vi "PH_Beckhoff_StepMot.set modified data.vi"(0 "i ref in":refnum<vi>, 2 "i attribute":T1, 5 "error in (no error)":errorcluster) -> (14 "i ref out":refnum<vi>, 19 "error out":errorcluster)   [LabVIEW 2014, in "PH_Beckhoff_StepMot.lvlib"]
doc: "Writes the data into the attribute of an object. Then, the attribute dara are unlocked using the \"release\" method. Prior to calling THIS method, the attribute data must have been locked using the methods \"lock\" or \"get data to modify\".\n\n\nLicense Agreement for this software:\n\nCopyright (C)\nGesellschaft für Schwerionenforschung, GSI\nPlanckstr. 1\n64291 Darmstadt\nGermany\n\nContact: D.Beck@gsi.de \n\nThis program is free software; you can redistribute it and/or modify it under the terms of the GNU General Public License as published by the Free Software Foundation; either version 2 of the license, or (at your option) any later version.\n\nThis program is distributed in the hope that it will be useful, but WITHOUT ANY WARRANTY; without even the implied warranty of MERCHANTABILITY or FITNESS FOR A PARTICULAR PURPOSE. See the GNU General License for more details (http://www.gnu.org).\n\nGesellschaft für Schwerionenforschung, GSI\nPlanckstr. 1, 64291 Darmstadt, Germany\nFor all questions and ideas contact: M.Richter@gsi.de, H.Brand@gsi.de or D.Beck@gsi.de.\nLast update: 17-JUN-2004"
uses:
  PH_Beckhoff_StepMot.lvlib
  PH_Beckhoff_StepMot.i attribute.ctl
  PH_Beckhoff_StepMot.Axis Cluster.ctl
  instr.lib/Beckhoff/Specials/Step Motor Klemmen/Beckhoff.Step Motor - Motor Configuration.ctl
  instr.lib/Beckhoff/Read and Write Register/Step Motor Klemmen/Beckhoff.Step Motor - Feature Register 1.ctl
  instr.lib/Beckhoff/Read and Write Register/Step Motor Klemmen/Beckhoff.Step Motor - Feature Register 2.ctl
  CS_Core/CSObj/CSObj.lvlib
  instr.lib/Beckhoff/Beckhoff - Driver np.lvlib
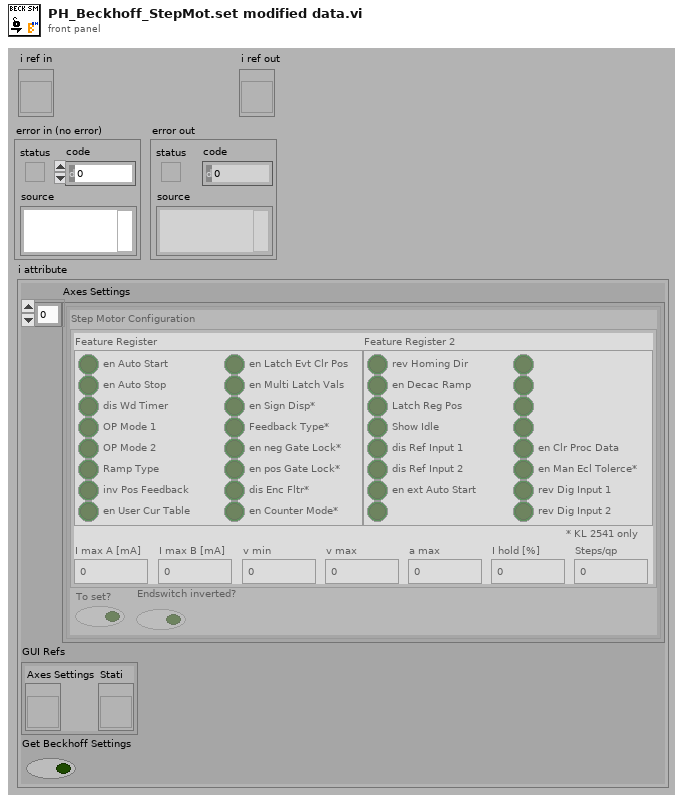
[diagram p1: front panel]
types:
  T1 = typedef "PH_Beckhoff_StepMot.lvlib/PH_Beckhoff_StepMot.i attribute.ctl" = cluster{"Axes Settings":T2[], "GUI Refs":cluster{"Axes Settings":refnum<vi>, "Stati":refnum<vi>}, "Get Beckhoff Settings":bool}
  T2 = typedef "PH_Beckhoff_StepMot.lvlib/PH_Beckhoff_StepMot.Axis Cluster.ctl" = cluster{"Step Motor Configuration":T3, "To set?":bool, "Endswitch inverted?":bool}
  T3 = typedef "Beckhoff - Driver np.lvlib/Beckhoff.Step Motor - Motor Configuration.ctl" = cluster{"Feature Register":T4, "I max A [mA]":dbl, "I max B [mA]":dbl, "v min":u32, "v max":u32, "a max":u32, "I hold [%]":u32, "Steps/qp":u32, "Feature Register 2":T5}
  T4 = typedef "Beckhoff - Driver np.lvlib/Beckhoff.Step Motor - Feature Register 1.ctl" = cluster{"en Auto Start":bool, "en Auto Stop":bool, "dis Wd Timer":bool, "OP Mode 1":bool, "OP Mode 2":bool, "Ramp Type":bool, "inv Pos Feedback":bool, "en User Cur Table":bool, "en Latch Evt Clr Pos":bool, "en Multi Latch Vals":bool, "en Sign Disp*":bool, "Feedback Type*":bool, "en neg Gate Lock*":bool, "en pos Gate Lock*":bool, "dis Enc Fltr*":bool, "en Counter Mode*":bool}
  T5 = typedef "Beckhoff - Driver np.lvlib/Beckhoff.Step Motor - Feature Register 2.ctl" = cluster{"rev Homing Dir":bool, "en Decac Ramp":bool, "Latch Reg Pos":bool, "Show Idle":bool, "dis Ref Input 1":bool, "dis Ref Input 2":bool, "en ext Auto Start":bool, "N/A":bool, "N/A":bool, "N/A":bool, "N/A":bool, "N/A":bool, "en Clr Proc Data":bool, "en Man Ecl Tolerce*":bool, "rev Dig Input 1":bool, "rev Dig Input 2":bool}
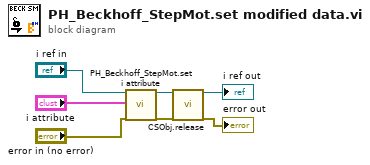
[diagram p0: block diagram]
diagram:
  n1 = call "PH_Beckhoff_StepMot.set i attribute.vi"("i ref in"="i ref in", "i attribute"="i attribute", "error in (no error)"="error in (no error)") -> ("i ref out"=w4:refnum<vi>, "error out"=w3:errorcluster)  [unwired: 15 in]
  n2 = call "CSObj.release.vi"("i ref in"=w4, "error in (no error)"=w3) -> ("i ref out"=→"i ref out":refnum<vi>, "error out"=→"error out":errorcluster)  [unwired: 16 in]
